vi "Version_4.9_8_on-chip_valves_for25ulSyringe_withModfied_Plunging.vi"() -> ()   [LabVIEW 2020] (continued)
                            n3174 = local read "VISA Refnum in\nfor Pump"() -> (w3578:refnum<visa-resource-name>)
                            n3175 = call "ProcessCompletionWaiter (SubVI).vi"("VISA Refnum in"=w3578) -> ()  [unwired: 11 in]
                          }
                          frame #2 {
                            # "If Yes, it will clean the elution buffer from port-5 tubing a bit more"
                            n3176 = local read "Clean the \nBuffer-B tubing"() -> (w3579:bool)
                            n3177 = case shown="True" w3579 {
                              frame False {
                                n3178 = stacked-sequence {
                                frame #0 {
                                n3179 = local read "Buffer-B Pumping\nResolution"() -> (w3582:T2)
                                n3180 = local read "VISA Refnum in\nfor Pump"() -> (w3584:refnum<visa-resource-name>)
                                n3181 = local read "V-S"() -> (w3581:dbl)
                                n3182 = local read "Volume of Syringe"() -> (w3583:dbl)
                                n3183 = call "RPickUp(SubVI).vi"("Volume to be picked up"=w3581, "Volume of Syringe"=w3583, "Resolution of PickUP"=w3582, "PickUp Flow Rate (ul/min)"=150.0, "VISA Refnum in"=w3584) -> ()  [unwired: 6 in, 1 out]
                                }
                                frame #1 {
                                n3184 = local read "Stopper that ends \nthe main loops"() -> (w3585:bool)
                                n3185 = local read "VISA Refnum in\nfor Pump"() -> (w3586:refnum<visa-resource-name>)
                                n3186 = case shown="True" w3585 {
                                frame False {
                                }
                                frame True {
                                n3187 = local read "VISA Refnum in\nfor Pump"() -> (w3587:refnum<visa-resource-name>)
                                n3188 = call "HardStopCurrentProcess (SubVI).vi"("VISA Refnum in"=w3587) -> ()  [unwired: 11 in]
                                }
                                }
                                n3189 = call "ProcessCompletionWaiter (SubVI).vi"("VISA Refnum in"=w3586) -> ()  [unwired: 11 in]
                                }
                                frame #2 {
                                n3190 = local read "VISA Refnum in\nfor Pump"() -> (w3589:refnum<visa-resource-name>)
                                n3191 = call "PortChanger (SubVI).vi"("Port Number"="1", "VISA Refnum in"=w3589) -> ()  [unwired: 10 in]
                                }
                                frame #3 {
                                n3192 = local read "Stopper that ends \nthe main loops"() -> (w3590:bool)
                                n3193 = local read "VISA Refnum in\nfor Pump"() -> (w3591:refnum<visa-resource-name>)
                                n3194 = case shown="True" w3590 {
                                frame False {
                                }
                                frame True {
                                n3195 = local read "VISA Refnum in\nfor Pump"() -> (w3592:refnum<visa-resource-name>)
                                n3196 = call "HardStopCurrentProcess (SubVI).vi"("VISA Refnum in"=w3592) -> ()  [unwired: 11 in]
                                }
                                }
                                n3197 = call "ProcessCompletionWaiter (SubVI).vi"("VISA Refnum in"=w3591) -> ()  [unwired: 11 in]
                                }
                                frame #4 {
                                n3198 = local read "VISA Refnum in\nfor Pump"() -> (w3597:refnum<visa-resource-name>)
                                n3199 = local read "Volume of Syringe"() -> (w3594:dbl)
                                n3200 = call "GoToAbsolutePosition(SubVI).vi"("Absolute Volume Position in Syringe (in ul)"=0.0, "Volume of Syringe"=w3594, "Resolution of Pumping"=T2."Standard Pumping", "Flow Rate (ul/min)"=150.0, "VISA Refnum in"=w3597) -> ()  [unwired: 6 in, 1 out]
                                }
                                frame #5 {
                                n3201 = local read "Stopper that ends \nthe main loops"() -> (w3598:bool)
                                n3202 = local read "VISA Refnum in\nfor Pump"() -> (w3599:refnum<visa-resource-name>)
                                n3203 = case shown="True" w3598 {
                                frame False {
                                }
                                frame True {
                                n3204 = local read "VISA Refnum in\nfor Pump"() -> (w3600:refnum<visa-resource-name>)
                                n3205 = call "HardStopCurrentProcess (SubVI).vi"("VISA Refnum in"=w3600) -> ()  [unwired: 11 in]
                                }
                                }
                                n3206 = call "ProcessCompletionWaiter (SubVI).vi"("VISA Refnum in"=w3599) -> ()  [unwired: 11 in]
                                }
                                }
                              }
                              frame True {
                                n3207 = for {
                                N: 2 -> [_]
                                n3208 = stacked-sequence {
                                frame #0 {
                                n3209 = local read "Buffer-B Pumping\nResolution"() -> (w3604:T2)
                                n3210 = local read "VISA Refnum in\nfor Pump"() -> (w3606:refnum<visa-resource-name>)
                                n3211 = local read "Apparent Volume\nof Syringe"() -> (w3603:dbl)
                                n3212 = local read "Volume of Syringe"() -> (w3605:dbl)
                                n3213 = call "RPickUp(SubVI).vi"("Volume to be picked up"=w3603, "Volume of Syringe"=w3605, "Resolution of PickUP"=w3604, "PickUp Flow Rate (ul/min)"=150.0, "VISA Refnum in"=w3606) -> ()  [unwired: 6 in, 1 out]
                                }
                                frame #1 {
                                n3214 = local read "Stopper that ends \nthe main loops"() -> (w3607:bool)
                                n3215 = local read "VISA Refnum in\nfor Pump"() -> (w3608:refnum<visa-resource-name>)
                                n3216 = case shown="True" w3607 {
                                frame False {
                                }
                                frame True {
                                n3217 = local read "VISA Refnum in\nfor Pump"() -> (w3609:refnum<visa-resource-name>)
                                n3218 = call "HardStopCurrentProcess (SubVI).vi"("VISA Refnum in"=w3609) -> ()  [unwired: 11 in]
                                }
                                }
                                n3219 = call "ProcessCompletionWaiter (SubVI).vi"("VISA Refnum in"=w3608) -> ()  [unwired: 11 in]
                                }
                                frame #2 {
                                n3220 = local read "VISA Refnum in\nfor Pump"() -> (w3611:refnum<visa-resource-name>)
                                n3221 = call "PortChanger (SubVI).vi"("Port Number"="1", "VISA Refnum in"=w3611) -> ()  [unwired: 10 in]
                                }
                                frame #3 {
                                n3222 = local read "Stopper that ends \nthe main loops"() -> (w3612:bool)
                                n3223 = local read "VISA Refnum in\nfor Pump"() -> (w3613:refnum<visa-resource-name>)
                                n3224 = case shown="True" w3612 {
                                frame False {
                                }
                                frame True {
                                n3225 = local read "VISA Refnum in\nfor Pump"() -> (w3614:refnum<visa-resource-name>)
                                n3226 = call "HardStopCurrentProcess (SubVI).vi"("VISA Refnum in"=w3614) -> ()  [unwired: 11 in]
                                }
                                }
                                n3227 = call "ProcessCompletionWaiter (SubVI).vi"("VISA Refnum in"=w3613) -> ()  [unwired: 11 in]
                                }
                                frame #4 {
                                n3228 = local read "VISA Refnum in\nfor Pump"() -> (w3619:refnum<visa-resource-name>)
                                n3229 = local read "Volume of Syringe"() -> (w3616:dbl)
                                n3230 = call "GoToAbsolutePosition(SubVI).vi"("Absolute Volume Position in Syringe (in ul)"=0.0, "Volume of Syringe"=w3616, "Resolution of Pumping"=T2."Standard Pumping", "Flow Rate (ul/min)"=150.0, "VISA Refnum in"=w3619) -> ()  [unwired: 6 in, 1 out]
                                }
                                frame #5 {
                                n3231 = local read "Stopper that ends \nthe main loops"() -> (w3620:bool)
                                n3232 = local read "VISA Refnum in\nfor Pump"() -> (w3621:refnum<visa-resource-name>)
                                n3233 = case shown="True" w3620 {
                                frame False {
                                }
                                frame True {
                                n3234 = local read "VISA Refnum in\nfor Pump"() -> (w3622:refnum<visa-resource-name>)
                                n3235 = call "HardStopCurrentProcess (SubVI).vi"("VISA Refnum in"=w3622) -> ()  [unwired: 11 in]
                                }
                                }
                                n3236 = call "ProcessCompletionWaiter (SubVI).vi"("VISA Refnum in"=w3621) -> ()  [unwired: 11 in]
                                }
                                }
                                }
                              }
                            }
                          }
                          frame #3 {
                            n3237 = local read "VISA Refnum in\nfor Pump"() -> (w3624:refnum<visa-resource-name>)
                            n3238 = local read "Port for \nB-Elution"() -> (w3623:string)
                            n3239 = call "PortChanger (SubVI).vi"("Port Number"=w3623, "VISA Refnum in"=w3624) -> ()  [unwired: 10 in]
                          }
                          frame #4 {
                            n3240 = local read "VISA Refnum in\nfor Pump"() -> (w3625:refnum<visa-resource-name>)
                            n3241 = call "ProcessCompletionWaiter (SubVI).vi"("VISA Refnum in"=w3625) -> ()  [unwired: 11 in]
                          }
                          frame #5 {
                            n3242 = local read "Buffer-B PickUp \nFlow Rate (ul/min)"() -> (w3628:dbl)
                            n3243 = local read "Buffer-B Pumping\nResolution"() -> (w3627:T2)
                            n3244 = local read "VISA Refnum in\nfor Pump"() -> (w3630:refnum<visa-resource-name>)
                            n3245 = local read "Buffer-B Volume \nto be  Pumped"() -> (w3626:dbl)
                            n3246 = local read "Volume of Syringe"() -> (w3629:dbl)
                            n3247 = call "RPickUp(SubVI).vi"("Volume to be picked up"=w3626, "Volume of Syringe"=w3629, "Resolution of PickUP"=w3627, "PickUp Flow Rate (ul/min)"=w3628, "VISA Refnum in"=w3630) -> ()  [unwired: 6 in, 1 out]
                          }
                          frame #6 {
                            n3248 = local read "Stopper that ends \nthe main loops"() -> (w3631:bool)
                            n3249 = local read "VISA Refnum in\nfor Pump"() -> (w3632:refnum<visa-resource-name>)
                            n3250 = case shown="True" w3631 {
                              frame False {
                              }
                              frame True {
                                n3251 = local read "VISA Refnum in\nfor Pump"() -> (w3633:refnum<visa-resource-name>)
                                n3252 = call "HardStopCurrentProcess (SubVI).vi"("VISA Refnum in"=w3633) -> ()  [unwired: 11 in]
                              }
                            }
                            n3253 = call "ProcessCompletionWaiter (SubVI).vi"("VISA Refnum in"=w3632) -> ()  [unwired: 11 in]
                          }
                          frame #7 {
                            # "Reads the initial Plunger Position for computing the volume dispensed"
                            n3254 = local read "VISA Refnum in\nfor Pump"() -> (w3635:refnum<visa-resource-name>)
                            n3255 = call "AbsolutePlungerPosition (SubVI).vi"("VISA Refnum in"=w3635) -> ("Plunger Position"=w3634:i32)  [unwired: 10 in]
                            n3256 = local write "Initial Plunger Position"(w3634) -> ()
                          }
                          frame #8 {
                            # "Switch to Port-2"
                            # "Port-2 of the pump is conncted to column-1 of chip"
                            n3257 = local read "VISA Refnum in\nfor Pump"() -> (w3637:refnum<visa-resource-name>)
                            n3258 = call "PortChanger (SubVI).vi"("Port Number"="2", "VISA Refnum in"=w3637) -> ()  [unwired: 10 in]
                          }
                          frame #9 {
                            n3259 = local read "Stopper that ends \nthe main loops"() -> (w3638:bool)
                            n3260 = local read "VISA Refnum in\nfor Pump"() -> (w3639:refnum<visa-resource-name>)
                            n3261 = case shown="True" w3638 {
                              frame False {
                              }
                              frame True {
                                n3262 = local read "VISA Refnum in\nfor Pump"() -> (w3640:refnum<visa-resource-name>)
                                n3263 = call "HardStopCurrentProcess (SubVI).vi"("VISA Refnum in"=w3640) -> ()  [unwired: 11 in]
                              }
                            }
                            n3264 = call "ProcessCompletionWaiter (SubVI).vi"("VISA Refnum in"=w3639) -> ()  [unwired: 11 in]
                          }
                          frame #10 {
                            # "Keeps the AMF valve after column-1 open and valve after column-2 closed"
                            n3265 = local read "VISA Refnum in\nfor Valve"() -> (w3645:refnum<visa-resource-name>)
                            n3266 = local read "External Valve \nOPEN"() -> (w3644:string)
                            n3267 = call "PortChanger_Valve (SubVI).vi"("Port Number"=w3644, "VISA Refnum in"=w3645) -> ()  [unwired: 10 in]
                            n3268 = local write "Valve V1 Open"(TRUE ("Valve V1 Open")) -> ()
                            n3269 = local write "Valve V2 Open"(TRUE ("Valve V2 Open")) -> ()
                            n3270 = local write "Valve V3 Open"(FALSE ("Valve V3 Open")) -> ()
                            n3271 = local write "Valve V4 Open"(FALSE ("Valve V4 Open")) -> ()
                            n3272 = local write "Valve V6 Open"(FALSE ("Valve V6 Open")) -> ()
                            n3273 = local write "Valve V5 Open"(FALSE ("Valve V5 Open")) -> ()
                            n3274 = local write "Valve V7 Open"(FALSE ("Valve V7 Open")) -> ()
                          }
                          frame #11 {
                            n3275 = local read "Buffer-B Dispense\nFlow Rate (ul/min)"() -> (w3655:dbl)
                            n3276 = local read "Buffer-B Pumping\nResolution"() -> (w3654:T2)
                            n3277 = local read "Initial Plunger Position"() -> (w3651:dbl)
                            n3278 = local read "VISA Refnum in\nfor Pump"() -> (w3657:refnum<visa-resource-name>)
                            n3279 = local read "Volume of Syringe"() -> (w3656:dbl)
                            n3280 = call "GoToAbsolutePosition(SubVI).vi"("Absolute Volume Position in Syringe (in ul)"=0.0 ("Volume to be Dispensed"), "Volume of Syringe"=w3656, "Resolution of Pumping"=w3654, "Flow Rate (ul/min)"=w3655, "VISA Refnum in"=w3657) -> ()  [unwired: 6 in, 1 out]
                            n3281 = local write "Pause Data Collection"(FALSE ("Pause Data Collection")) -> ()
                            n3282 = local write "Vol_now"(0.0 ("Vol_now")) -> ()
                            n3283 = local write "Position\nNow"(w3651) -> ()
                          }
                          frame #12 {
                            n3284 = while {
                              stop <- w3664 stop-if-true
                              n3285 = event shown="[0] \"Pause Elution Value\": Value Change" {
                                selector: _ -> [_ _]
                                dyn-events: _ -> [_ _]
                                timeout: 100 -> [_ _]
                                event "Pause Elution\nValue": Value Change {
                                n3286 = event-data() -> ()  [unwired: 1 in, 6 out]
                                n3287 = stacked-sequence {
                                frame #0 {
                                n3288 = local read "Pause Elution"() -> (w3666:bool)
                                n3289 = case shown="False" w3666 {
                                frame False {
                                n3290 = local write "Pause Elution"(TRUE ("Pause Elution")) -> ()
                                }
                                frame True {
                                n3291 = local write "Pause Elution"(FALSE ("Pause Elution")) -> ()
                                }
                                }
                                }
                                frame #1 {
                                n3292 = local read "Pause Elution"() -> (w3669:bool)
                                n3293 = case shown="False" w3669 {
                                frame False {
                                n3294 = local read "Buffer-B Dispense\nFlow Rate (ul/min)"() -> (w3674:dbl)
                                n3295 = local read "VISA Refnum in\nfor Pump"() -> (w3675:refnum<visa-resource-name>)
                                n3296 = local read "Buffer-B Pumping\nResolution"() -> (w3671:T2)
                                n3297 = local read "Volume of Syringe"() -> (w3672:dbl)
                                n3298 = call "GoToAbsolutePosition(SubVI).vi"("Absolute Volume Position in Syringe (in ul)"=0.0, "Volume of Syringe"=w3672, "Resolution of Pumping"=w3671, "Flow Rate (ul/min)"=w3674, "VISA Refnum in"=w3675) -> ()  [unwired: 6 in, 1 out]
                                n3299 = local write "Pause Data Collection"(FALSE ("Pause Data Collection")) -> ()
                                }
                                frame True {
                                n3300 = local read "VISA Refnum in\nfor Pump"() -> (w3677:refnum<visa-resource-name>)
                                n3301 = local write "Pause Data Collection"(TRUE ("Pause Data Collection")) -> ()
                                n3302 = call "HardStopCurrentProcess (SubVI).vi"("VISA Refnum in"=w3677) -> ()  [unwired: 11 in]
                                }
                                }
                                }
                                }
                                }
                                event Timeout {
                                n3303 = event-data() -> ()  [unwired: 1 in, 3 out]
                                }
                              }
                              n3304 = local read "Divert Sample \ninto Column-2"() -> (w3663:bool)
                              n3305 = local read "Stopper that ends \nthe main loops"() -> (w3662:bool)
                              n3306 = Or(x=w3663, y=w3662) -> (x .or. y?=w3664:bool)
                            }
                            n3307 = local read "Buffer-B Pumping\nResolution"() -> (w3660:T2)
                            n3308 = local read "VISA Refnum in\nfor Pump"() -> (w3661:refnum<visa-resource-name>)
                            n3309 = local read "Volume of Syringe"() -> (w3659:dbl)
                            n3310 = while {
                              tunnel: w3661 -> [w3686]
                              tunnel: w3660 -> [w3685]
                              tunnel: w3659 -> [w3684]
                              stop <- w3680 stop-if-true
                              n3311 = local read "Position\nNow"() -> (w3678:dbl)
                              n3312 = local read "Pause Elution"() -> (w3679:bool)
                              n3313 = case shown="True" w3679 {
                                tunnel: w3678 -> [w3690 _]
                                tunnel: w3686 -> [w3689 w3732]
                                tunnel: w3685 -> [w3688 _]
                                tunnel: w3684 -> [w3687 _]
                                frame False {
                                n3314 = stacked-sequence {
                                tunnel: w3690 -> [_ w3696]
                                tunnel: w3689 -> [_ w3695]
                                tunnel: w3688 -> [_ w3694]
                                tunnel: w3687 -> [_ w3693]
                                frame #0 {
                                n3315 = Wait (ms)(milliseconds to wait=u32 3000) -> ()  [unwired: 1 out]
                                n3316 = local write "Signal"(TRUE ("Signal")) -> ()
                                }
                                frame #1 {
                                n3317 = while {
                                tunnel: w3696 -> [w3708]
                                tunnel: w3695 -> [w3707]
                                tunnel: w3694 -> [w3706]
                                tunnel: w3693 -> [w3705]
                                stop <- w3700 stop-if-true
                                n3318 = stacked-sequence {
                                tunnel: w3708 -> [_ w3715]
                                tunnel: w3707 -> [_ w3714]
                                tunnel: w3706 -> [_ w3713]
                                tunnel: w3705 -> [_ w3712]
                                frame #0 {
                                n3319 = Wait (ms)(milliseconds to wait=u32 500) -> ()  [unwired: 1 out]
                                }
                                frame #1 {
                                n3320 = call "AbsolutePlungerPosition (SubVI).vi"("VISA Refnum in"=w3714) -> ("Plunger Position"=w3711:i32)  [unwired: 10 in]
                                n3321 = case shown="\"High Resolution Pumping\"" w3713 {
                                tunnel: w3715 -> [w3720 w3729]
                                tunnel: w3711 -> [w3721 w3728]
                                tunnel: [w3719 w3726] -> w3710
                                tunnel: w3712 -> [w3718 w3727]
                                frame "Standard Pumping", Default {
                                n3322 = Subtract(x=w3720, y=w3721) -> (x-y=w3717:dbl)
                                n3323 = Absolute Value(x=w3717) -> (abs(x)=w3716:dbl)
                                n3324 = Multiply(x=w3716, y=w3718) -> (x*y=w3723:dbl)
                                n3325 = Divide(x=w3723, y=3000.0) -> (x/y=w3719:dbl)
                                }
                                frame "High Resolution Pumping" {
                                n3326 = Subtract(x=w3729, y=w3728) -> (x-y=w3725:dbl)
                                n3327 = Absolute Value(x=w3725) -> (abs(x)=w3724:dbl)
                                n3328 = Multiply(x=w3724, y=w3727) -> (x*y=w3731:dbl)
                                n3329 = Divide(x=w3731, y=24000.0) -> (x/y=w3726:dbl)
                                }
                                }
                                n3330 = local write "Volume being Injected \nin this process"(w3710) -> ()
                                }
                                }
                                n3331 = local read "Volume being Injected \nin this process"() -> (w3698:dbl)
                                n3332 = local read "Affinity Elution \nGraph Min CutOff"() -> (w3697:dbl)
                                n3333 = local read "Stopper that ends \nthe main loops"() -> (w3703:bool)
                                n3334 = local read "Divert Sample \ninto Column-2"() -> (w3704:bool)
                                n3335 = Greater Or Equal?(x=w3698, y=w3697) -> (x >= y?=w3699:bool)
                                n3336 = Or(x=w3704, y=w3703) -> (x .or. y?=w3701:bool)
                                n3337 = local read "Pause Elution"() -> (w3702:bool)
                                n3338 = local write "Affinity Elution \nis Approaching"(w3699) -> ()
                                n3339 = Or(x=w3702, y=w3701) -> (x .or. y?=w3700:bool)
                                }
                                }
                                }
                                }
                                frame True {
                                n3340 = stacked-sequence {
                                tunnel: w3732 -> [_ w3735 _]
                                frame #0 {
                                n3341 = Wait (ms)(milliseconds to wait=u32 2000) -> ()  [unwired: 1 out]
                                }
                                frame #1 {
                                n3342 = local read "Signal"() -> (w3734:bool)
                                n3343 = case shown="True" w3734 {
                                tunnel: w3735 -> [_ w3741]
                                frame False {
                                }
                                frame True {
                                n3344 = local read "Volume being Injected \nin this process"() -> (w3739:dbl)
                                n3345 = local read "Net Elution \nVolume"() -> (w3738:dbl)
                                n3346 = local write "Signal"(FALSE ("Signal")) -> ()
                                n3347 = Add(x=w3739, y=w3738) -> (x+y=w3737:dbl)
                                n3348 = call "AbsolutePlungerPosition (SubVI).vi"("VISA Refnum in"=w3741) -> ("Plunger Position"=w3740:i32)  [unwired: 10 in]
                                n3349 = local write "Net Elution \nVolume"(w3737) -> ()
                                n3350 = local write "Position\nNow"(w3740) -> ()
                                }
                                }
                                }
                                frame #2 {
                                n3351 = local write "Volume being Injected \nin this process"(0.0 ("Volume being Injected \nin this process")) -> ()
                                }
                                }
                                }
                              }
                              n3352 = local read "Stopper that ends \nthe main loops"() -> (w3682:bool)
                              n3353 = local read "Divert Sample \ninto Column-2"() -> (w3681:bool)
                              n3354 = Or(x=w3681, y=w3682) -> (x .or. y?=w3680:bool)
                              n3355 = Wait (ms)(milliseconds to wait=u32 300) -> ()  [unwired: 1 out]
                            }
                            n3356 = local read "Stopper that ends \nthe main loops"() -> (w3658:bool)
                            n3357 = case shown="True" w3658 {
                              frame False {
                              }
                              frame True {
                                n3358 = local read "VISA Refnum in\nfor Pump"() -> (w3743:refnum<visa-resource-name>)
                                n3359 = call "HardStopCurrentProcess (SubVI).vi"("VISA Refnum in"=w3743) -> ()  [unwired: 11 in]
                              }
                            }
                          }
                          frame #13 {
                            # "valve after column-1 is closed"
                            # "Keeps the on-chip Valve V1 and V3 after column-2 open"
                            # "Keeps the AMF valve after column-1 closed and valve after column-2 open"
                            n3360 = local read "VISA Refnum in\nfor Pump"() -> (w3756:refnum<visa-resource-name>)
                            n3361 = local read "Volume being Injected \nin this process"() -> (w3753:dbl)
                            n3362 = local write "Sample Volume Diverted\ninto Column-2"(0.0 ("Sample Volume Diverted\ninto Column-2")) -> ()
                            n3363 = call "AbsolutePlungerPosition (SubVI).vi"("VISA Refnum in"=w3756) -> ("Plunger Position"=w3755:i32)  [unwired: 10 in]
                            n3364 = local write "Position\nNow"(w3755) -> ()
                            n3365 = local write "Vol_previous"(0.0 ("Vol_diff")) -> ()
                            n3366 = local write "Vol_now"(w3753) -> ()
                            n3367 = local read "VISA Refnum in\nfor Valve"() -> (w3748:refnum<visa-resource-name>)
                            n3368 = local read "External Valve \nCLOSED"() -> (w3747:string)
                            n3369 = local write "Valve V1 Open"(TRUE ("Valve V1 Open")) -> ()
                            n3370 = local write "Valve V3 Open"(TRUE ("Valve V3 Open")) -> ()
                            n3371 = local write "Valve V2 Open"(FALSE ("Valve V2 Open")) -> ()
                            n3372 = local write "Valve V4 Open"(TRUE ("Valve V4 Open")) -> ()
                            n3373 = call "PortChanger_Valve (SubVI).vi"("Port Number"=w3747, "VISA Refnum in"=w3748) -> ()  [unwired: 10 in]
                            n3374 = local write "Valve V5 Open"(TRUE ("Valve V5 Open")) -> ()
                            n3375 = local write "Valve V6 Open"(FALSE ("Valve V6 Open")) -> ()
                            n3376 = local write "Valve V7 Open"(TRUE ("Valve V7 Open")) -> ()
                          }
                          frame #14 {
                            n3377 = local read "Divert Sample \ninto Column-2"() -> (w3758:bool)
                            n3378 = case shown="True" w3758 {
                              frame False {
                                n3379 = stacked-sequence {
                                frame #0 {
                                n3380 = local read "Buffer-B Pumping\nResolution"() -> (w3761:T2)
                                n3381 = local read "VISA Refnum in\nfor Pump"() -> (w3763:refnum<visa-resource-name>)
                                n3382 = local read "Initial Plunger Position"() -> (w3762:dbl)
                                n3383 = local read "Volume of Syringe"() -> (w3760:dbl)
                                n3384 = while {
                                tunnel: w3762 -> [w3769]
                                tunnel: w3763 -> [w3768]
                                tunnel: w3761 -> [w3767]
                                tunnel: w3760 -> [w3766]
                                stop <- w3764 stop-if-true
                                n3385 = Wait (ms)(milliseconds to wait=u32 100) -> ()  [unwired: 1 out]
                                n3386 = stacked-sequence {
                                tunnel: w3769 -> [w3775 _]
                                tunnel: w3768 -> [w3774 w3795]
                                tunnel: w3767 -> [w3773 _]
                                tunnel: w3766 -> [w3772 _]
                                tunnel: [_ w3793] -> w3764
                                frame #0 {
                                n3387 = call "AbsolutePlungerPosition (SubVI).vi"("VISA Refnum in"=w3774) -> ("Plunger Position"=w3771:i32)  [unwired: 10 in]
                                n3388 = case shown="\"Standard Pumping\", Default" w3773 {
                                tunnel: w3775 -> [w3780 w3789]
                                tunnel: w3771 -> [w3781 w3788]
                                tunnel: [w3779 w3786] -> w3770
                                tunnel: w3772 -> [w3778 w3787]
                                frame "Standard Pumping", Default {
                                n3389 = Subtract(x=w3780, y=w3781) -> (x-y=w3777:dbl)
                                n3390 = Absolute Value(x=w3777) -> (abs(x)=w3776:dbl)
                                n3391 = Multiply(x=w3776, y=w3778) -> (x*y=w3783:dbl)
                                n3392 = Divide(x=w3783, y=3000.0) -> (x/y=w3779:dbl)
                                }
                                frame "High Resolution Pumping" {
                                n3393 = Subtract(x=w3789, y=w3788) -> (x-y=w3785:dbl)
                                n3394 = Absolute Value(x=w3785) -> (abs(x)=w3784:dbl)
                                n3395 = Multiply(x=w3784, y=w3787) -> (x*y=w3791:dbl)
                                n3396 = Divide(x=w3791, y=24000.0) -> (x/y=w3786:dbl)
                                }
                                }
                                n3397 = local write "Volume being Injected \nin this process"(w3770) -> ()
                                }
                                frame #1 {
                                n3398 = local read "Stopper that ends \nthe main loops"() -> (w3792:bool)
                                n3399 = call "LSPOneStatus (SubVI).vi"("VISA Refnum in"=w3795) -> ("read buffer"=w3797:string)  [unwired: 10 in]
                                n3400 = call <vilib>:"Trim Whitespace.vi"("string"=w3797) -> ("trimmed string"=w3796:string)  [unwired: 1 in]
                                n3401 = Equal?(x=w3796, y="/0`\u0003") -> (x = y?=w3794:bool)
                                n3402 = Or(x=w3794, y=w3792) -> (x .or. y?=w3793:bool)
                                }
                                }
                                }
                                n3403 = local read "Stopper that ends \nthe main loops"() -> (w3759:bool)
                                n3404 = case shown="True" w3759 {
                                frame False {
                                }
                                frame True {
                                n3405 = local read "VISA Refnum in\nfor Pump"() -> (w3799:refnum<visa-resource-name>)
                                n3406 = call "HardStopCurrentProcess (SubVI).vi"("VISA Refnum in"=w3799) -> ()  [unwired: 11 in]
                                }
                                }
                                }
                                }
                              }
                              frame True {
                                n3407 = stacked-sequence {
                                frame #0 {
                                n3408 = local read "Buffer-B Pumping\nResolution"() -> (w3802:T2)
                                n3409 = local read "VISA Refnum in\nfor Pump"() -> (w3804:refnum<visa-resource-name>)
                                n3410 = local read "Volume of Syringe"() -> (w3801:dbl)
                                n3411 = local read "Position\nNow"() -> (w3803:dbl)
                                n3412 = while {
                                tunnel: w3803 -> [w3810]
                                tunnel: w3804 -> [w3809]
                                tunnel: w3802 -> [w3808]
                                tunnel: w3801 -> [w3807]
                                stop <- w3805 stop-if-true
                                n3413 = Wait (ms)(milliseconds to wait=u32 100) -> ()  [unwired: 1 out]
                                n3414 = stacked-sequence {
                                tunnel: w3810 -> [w3820 _ _]
                                tunnel: w3809 -> [w3819 _ w3846]
                                tunnel: w3808 -> [w3818 _ _]
                                tunnel: w3807 -> [w3817 _ _]
                                tunnel: [_ _ w3844] -> w3805
                                frame #0 {
                                n3415 = local read "Vol_previous"() -> (w3814:dbl)
                                n3416 = call "AbsolutePlungerPosition (SubVI).vi"("VISA Refnum in"=w3819) -> ("Plunger Position"=w3816:i32)  [unwired: 10 in]
                                n3417 = case shown="\"Standard Pumping\", Default" w3818 {
                                tunnel: w3820 -> [w3825 w3834]
                                tunnel: w3816 -> [w3826 w3833]
                                tunnel: [w3824 w3831] -> w3815
                                tunnel: w3817 -> [w3823 w3832]
                                frame "Standard Pumping", Default {
                                n3418 = Subtract(x=w3825, y=w3826) -> (x-y=w3822:dbl)
                                n3419 = Absolute Value(x=w3822) -> (abs(x)=w3821:dbl)
                                n3420 = Multiply(x=w3821, y=w3823) -> (x*y=w3828:dbl)
                                n3421 = Divide(x=w3828, y=3000.0) -> (x/y=w3824:dbl)
                                }
                                frame "High Resolution Pumping" {
                                n3422 = Subtract(x=w3834, y=w3833) -> (x-y=w3830:dbl)
                                n3423 = Absolute Value(x=w3830) -> (abs(x)=w3829:dbl)
                                n3424 = Multiply(x=w3829, y=w3832) -> (x*y=w3836:dbl)
                                n3425 = Divide(x=w3836, y=24000.0) -> (x/y=w3831:dbl)
                                }
                                }
                                n3426 = Subtract(x=w3815, y=w3814) -> (x-y=w3813:dbl)
                                n3427 = local read "Vol_now"() -> (w3811:dbl)
                                n3428 = local write "Sample Volume Diverted\ninto Column-2"(w3815) -> ()
                                n3429 = Add(x=w3813, y=w3811) -> (x+y=w3812:dbl)
                                n3430 = local write "Volume being Injected \nin this process"(w3812) -> ()
                                }
                                frame #1 {
                                n3431 = local read "Volume being Injected \nin this process"() -> (w3837:dbl)
                                n3432 = local read "Sample Volume Diverted\ninto Column-2"() -> (w3838:dbl)
                                n3433 = local write "Vol_now"(w3837) -> ()
                                n3434 = local write "Vol_previous"(w3838) -> ()
                                }
                                frame #2 {
                                n3435 = local read "Buffer-B Volume \nto be Pumped for\nSample Diversion\nto Column-2"() -> (w3840:dbl)
                                n3436 = local read "Sample Volume Diverted\ninto Column-2"() -> (w3839:dbl)
                                n3437 = local read "Stopper that ends \nthe main loops"() -> (w3841:bool)
                                n3438 = call "LSPOneStatus (SubVI).vi"("VISA Refnum in"=w3846) -> ("read buffer"=w3848:string)  [unwired: 10 in]
                                n3439 = call <vilib>:"Trim Whitespace.vi"("string"=w3848) -> ("trimmed string"=w3847:string)  [unwired: 1 in]
                                n3440 = Equal?(x=w3847, y="/0`\u0003") -> (x = y?=w3845:bool)
                                n3441 = Greater Or Equal?(x=w3839, y=w3840) -> (x >= y?=w3843:bool)
                                n3442 = Or(x=w3841, y=w3843) -> (x .or. y?=w3842:bool)
                                n3443 = Or(x=w3845, y=w3842) -> (x .or. y?=w3844:bool)
                                }
                                }
                                }
                                n3444 = local read "Stopper that ends \nthe main loops"() -> (w3800:bool)
                                n3445 = case shown="True" w3800 {
                                frame False {
                                }
                                frame True {
                                n3446 = local read "VISA Refnum in\nfor Pump"() -> (w3850:refnum<visa-resource-name>)
                                n3447 = call "HardStopCurrentProcess (SubVI).vi"("VISA Refnum in"=w3850) -> ()  [unwired: 11 in]
                                }
                                }
                                }
                                frame #1 {
                                n3448 = local read "VISA Refnum in\nfor Pump"() -> (w3852:refnum<visa-resource-name>)
                                n3449 = local write "Pause Data Collection"(TRUE ("Pause Data Collection")) -> ()
                                n3450 = call "HardStopCurrentProcess (SubVI).vi"("VISA Refnum in"=w3852) -> ()  [unwired: 11 in]
                                }
                                frame #2 {
                                n3451 = local read "VISA Refnum in\nfor Pump"() -> (w3853:refnum<visa-resource-name>)
                                n3452 = call "PortChanger (SubVI).vi"("Port Number"="1", "VISA Refnum in"=w3853) -> ()  [unwired: 10 in]
                                }
                                frame #3 {
                                n3453 = local read "VISA Refnum in\nfor Pump"() -> (w3859:refnum<visa-resource-name>)
                                n3454 = local read "Volume of Syringe"() -> (w3855:dbl)
                                n3455 = call "GoToAbsolutePosition(SubVI).vi"("Absolute Volume Position in Syringe (in ul)"=0.0, "Volume of Syringe"=w3855, "Resolution of Pumping"=T2."Standard Pumping", "Flow Rate (ul/min)"=150.0, "VISA Refnum in"=w3859) -> ()  [unwired: 6 in, 1 out]
                                }
                                frame #4 {
                                n3456 = local read "VISA Refnum in\nfor Pump"() -> (w3861:refnum<visa-resource-name>)
                                n3457 = local write "Divert Sample \ninto Column-2"(FALSE ("Divert Sample \ninto Column-2")) -> ()
                                n3458 = call "ProcessCompletionWaiter (SubVI).vi"("VISA Refnum in"=w3861) -> ()  [unwired: 11 in]
                                }
                                }
                              }
                            }
                          }
                          frame #15 {
                            # "Keeps the On-Chip Valves V1 and V3 closed"
                            # "Switch to Port-5/8"
                            # "Port-5/8 of pump is connected to Buffer-C1/C2"
                            # "Keeps the AMF valve after column-1 open and valve after column-2 closed"
                            n3459 = local read "VISA Refnum in\nfor Pump"() -> (w3874:refnum<visa-resource-name>)
                            n3460 = local write "Pause Data Collection"(TRUE ("Pause Data Collection")) -> ()
                            n3461 = Wait (ms)(milliseconds to wait=u32 500) -> ()  [unwired: 1 out]
                            n3462 = local write "Affinity On"(FALSE ("Affinity On")) -> ()
                            n3463 = local read "Port for \nC2-Elution"() -> (w3865:string)
                            n3464 = local write "Affinity Elution On"(FALSE ("Affinity Elution On")) -> ()
                            n3465 = call "PortChanger (SubVI).vi"("Port Number"=w3865, "VISA Refnum in"=w3874) -> ()  [unwired: 10 in]
                            n3466 = local read "VISA Refnum in\nfor Valve"() -> (w3868:refnum<visa-resource-name>)
                            n3467 = local read "External Valve \nCLOSED"() -> (w3867:string)
                            n3468 = local write "Valve V1 Open"(FALSE ("Valve V1 Open")) -> ()
                            n3469 = local write "Valve V2 Open"(FALSE ("Valve V2 Open")) -> ()
                            n3470 = local write "Valve V3 Open"(FALSE ("Valve V3 Open")) -> ()
                            n3471 = local write "Valve V4 Open"(FALSE ("Valve V4 Open")) -> ()
                            n3472 = call "PortChanger_Valve (SubVI).vi"("Port Number"=w3867, "VISA Refnum in"=w3868) -> ()  [unwired: 10 in]
                            n3473 = local write "Valve V5 Open"(FALSE ("Valve V5 Open")) -> ()
                            n3474 = local write "Valve V6 Open"(FALSE ("Valve V6 Open")) -> ()
                            n3475 = local write "Valve V7 Open"(FALSE ("Valve V7 Open")) -> ()
                          }
                          frame #16 {
                            n3476 = local read "VISA Refnum in\nfor Pump"() -> (w3878:refnum<visa-resource-name>)
                            n3477 = call "ProcessCompletionWaiter (SubVI).vi"("VISA Refnum in"=w3878) -> ()  [unwired: 11 in]
                            n3478 = local write "Start the Process"(FALSE ("Start the Process")) -> ()
                          }
                          frame #17 {
                            n3479 = local read "Stopper that ends \nthe main loops"() -> (w3882:bool)
                            n3480 = local read "Start the Process"() -> (w3883:bool)
                            n3481 = Or(x=w3883, y=w3882) -> (x .or. y?=w3881:bool)
                            n3482 = local write "Elution of Column-1"(FALSE ("Elution of Column-1")) -> ()
                            n3483 = case shown="False" w3881 {
                              frame False {
                                n3484 = while {
                                stop <- w3887 stop-if-true
                                n3485 = local read "Stopper that ends \nthe main loops"() -> (w3888:bool)
                                n3486 = local read "Start the Process"() -> (w3889:bool)
                                n3487 = Or(x=w3889, y=w3888) -> (x .or. y?=w3887:bool)
                                n3488 = Wait (ms)(milliseconds to wait=u32 10) -> ()  [unwired: 1 out]
                                }
                                n3489 = One Button Dialog(message="Move to Column-2 detection zone and Press 'Start the Process' Button.") -> ()  [unwired: 1 in, 1 out]
                              }
                              frame True {
                              }
                            }
                            n3490 = local write "Volume being Injected \nin this process"(0.0 ("Volume being Injected \nin this process")) -> ()
                            n3491 = local write "Elution of Column-2"(TRUE ("Elution of Column-2")) -> ()
                          }
                          frame #18 {
                            # "If Yes, it will clean the SEC buffer from port-8 tubing else it will clean the pump valve a bit"
                            n3492 = local read "Clean the \nBuffer-C2 tubing"() -> (w3890:bool)
                            n3493 = case shown="False" w3890 {
                              frame False {
                                n3494 = stacked-sequence {
                                frame #0 {
                                n3495 = local read "VISA Refnum in\nfor Pump"() -> (w3892:refnum<visa-resource-name>)
                                n3496 = local read "Port for \nC2-Elution"() -> (w3891:string)
                                n3497 = call "PortChanger (SubVI).vi"("Port Number"=w3891, "VISA Refnum in"=w3892) -> ()  [unwired: 10 in]
                                }
                                frame #1 {
                                n3498 = local read "VISA Refnum in\nfor Pump"() -> (w3893:refnum<visa-resource-name>)
                                n3499 = call "ProcessCompletionWaiter (SubVI).vi"("VISA Refnum in"=w3893) -> ()  [unwired: 11 in]
                                }
                                frame #2 {
                                n3500 = local read "Buffer-C2 Pumping\nResolution"() -> (w3896:T2)
                                n3501 = local read "VISA Refnum in\nfor Pump"() -> (w3898:refnum<visa-resource-name>)
                                n3502 = local read "V-S"() -> (w3894:dbl)
                                n3503 = local read "Volume of Syringe"() -> (w3897:dbl)
                                n3504 = call "RPickUp(SubVI).vi"("Volume to be picked up"=w3894, "Volume of Syringe"=w3897, "Resolution of PickUP"=w3896, "PickUp Flow Rate (ul/min)"=150.0, "VISA Refnum in"=w3898) -> ()  [unwired: 6 in, 1 out]
                                }
                                frame #3 {
                                n3505 = local read "Stopper that ends \nthe main loops"() -> (w3899:bool)
                                n3506 = local read "VISA Refnum in\nfor Pump"() -> (w3900:refnum<visa-resource-name>)
                                n3507 = case shown="True" w3899 {
                                frame False {
                                }
                                frame True {
                                n3508 = local read "VISA Refnum in\nfor Pump"() -> (w3901:refnum<visa-resource-name>)
                                n3509 = call "HardStopCurrentProcess (SubVI).vi"("VISA Refnum in"=w3901) -> ()  [unwired: 11 in]
                                }
                                }
                                n3510 = call "ProcessCompletionWaiter (SubVI).vi"("VISA Refnum in"=w3900) -> ()  [unwired: 11 in]
                                }
                                frame #4 {
                                n3511 = local read "VISA Refnum in\nfor Pump"() -> (w3903:refnum<visa-resource-name>)
                                n3512 = call "PortChanger (SubVI).vi"("Port Number"="1", "VISA Refnum in"=w3903) -> ()  [unwired: 10 in]
                                }
                                frame #5 {
                                n3513 = local read "Stopper that ends \nthe main loops"() -> (w3904:bool)
                                n3514 = local read "VISA Refnum in\nfor Pump"() -> (w3905:refnum<visa-resource-name>)
                                n3515 = case shown="True" w3904 {
                                frame False {
                                }
                                frame True {
                                n3516 = local read "VISA Refnum in\nfor Pump"() -> (w3906:refnum<visa-resource-name>)
                                n3517 = call "HardStopCurrentProcess (SubVI).vi"("VISA Refnum in"=w3906) -> ()  [unwired: 11 in]
                                }
                                }
                                n3518 = call "ProcessCompletionWaiter (SubVI).vi"("VISA Refnum in"=w3905) -> ()  [unwired: 11 in]
                                }
                                frame #6 {
                                n3519 = local read "VISA Refnum in\nfor Pump"() -> (w3911:refnum<visa-resource-name>)
                                n3520 = local read "Volume of Syringe"() -> (w3908:dbl)
                                n3521 = call "GoToAbsolutePosition(SubVI).vi"("Absolute Volume Position in Syringe (in ul)"=0.0, "Volume of Syringe"=w3908, "Resolution of Pumping"=T2."Standard Pumping", "Flow Rate (ul/min)"=150.0, "VISA Refnum in"=w3911) -> ()  [unwired: 6 in, 1 out]
                                }
                                frame #7 {
                                n3522 = local read "Stopper that ends \nthe main loops"() -> (w3912:bool)
                                n3523 = local read "VISA Refnum in\nfor Pump"() -> (w3913:refnum<visa-resource-name>)
                                n3524 = case shown="True" w3912 {
                                frame False {
                                }
                                frame True {
                                n3525 = local read "VISA Refnum in\nfor Pump"() -> (w3914:refnum<visa-resource-name>)
                                n3526 = call "HardStopCurrentProcess (SubVI).vi"("VISA Refnum in"=w3914) -> ()  [unwired: 11 in]
                                }
                                }
                                n3527 = call "ProcessCompletionWaiter (SubVI).vi"("VISA Refnum in"=w3913) -> ()  [unwired: 11 in]
                                }
                                }
                              }
                              frame True {
                                n3528 = for {
                                N: 2 -> [_]
                                n3529 = stacked-sequence {
                                frame #0 {
                                n3530 = local read "VISA Refnum in\nfor Pump"() -> (w3917:refnum<visa-resource-name>)
                                n3531 = local read "Port for \nC2-Elution"() -> (w3916:string)
                                n3532 = call "PortChanger (SubVI).vi"("Port Number"=w3916, "VISA Refnum in"=w3917) -> ()  [unwired: 10 in]
                                }
                                frame #1 {
                                n3533 = local read "VISA Refnum in\nfor Pump"() -> (w3918:refnum<visa-resource-name>)
                                n3534 = call "ProcessCompletionWaiter (SubVI).vi"("VISA Refnum in"=w3918) -> ()  [unwired: 11 in]
                                }
                                frame #2 {
                                n3535 = local read "Buffer-C2 Pumping\nResolution"() -> (w3921:T2)
                                n3536 = local read "VISA Refnum in\nfor Pump"() -> (w3923:refnum<visa-resource-name>)
                                n3537 = local read "Apparent Volume\nof Syringe"() -> (w3919:dbl)
                                n3538 = local read "Volume of Syringe"() -> (w3922:dbl)
                                n3539 = call "RPickUp(SubVI).vi"("Volume to be picked up"=w3919, "Volume of Syringe"=w3922, "Resolution of PickUP"=w3921, "PickUp Flow Rate (ul/min)"=150.0, "VISA Refnum in"=w3923) -> ()  [unwired: 6 in, 1 out]
                                }
                                frame #3 {
                                n3540 = local read "Stopper that ends \nthe main loops"() -> (w3924:bool)
                                n3541 = local read "VISA Refnum in\nfor Pump"() -> (w3925:refnum<visa-resource-name>)
                                n3542 = case shown="True" w3924 {
                                frame False {
                                }
                                frame True {
                                n3543 = local read "VISA Refnum in\nfor Pump"() -> (w3926:refnum<visa-resource-name>)
                                n3544 = call "HardStopCurrentProcess (SubVI).vi"("VISA Refnum in"=w3926) -> ()  [unwired: 11 in]
                                }
                                }
                                n3545 = call "ProcessCompletionWaiter (SubVI).vi"("VISA Refnum in"=w3925) -> ()  [unwired: 11 in]
                                }
                                frame #4 {
                                n3546 = local read "VISA Refnum in\nfor Pump"() -> (w3928:refnum<visa-resource-name>)
                                n3547 = call "PortChanger (SubVI).vi"("Port Number"="1", "VISA Refnum in"=w3928) -> ()  [unwired: 10 in]
                                }
                                frame #5 {
                                n3548 = local read "Stopper that ends \nthe main loops"() -> (w3929:bool)
                                n3549 = local read "VISA Refnum in\nfor Pump"() -> (w3930:refnum<visa-resource-name>)
                                n3550 = case shown="True" w3929 {
                                frame False {
                                }
                                frame True {
                                n3551 = local read "VISA Refnum in\nfor Pump"() -> (w3931:refnum<visa-resource-name>)
                                n3552 = call "HardStopCurrentProcess (SubVI).vi"("VISA Refnum in"=w3931) -> ()  [unwired: 11 in]
                                }
                                }
                                n3553 = call "ProcessCompletionWaiter (SubVI).vi"("VISA Refnum in"=w3930) -> ()  [unwired: 11 in]
                                }
                                frame #6 {
                                n3554 = local read "VISA Refnum in\nfor Pump"() -> (w3936:refnum<visa-resource-name>)
                                n3555 = local read "Volume of Syringe"() -> (w3933:dbl)
                                n3556 = call "GoToAbsolutePosition(SubVI).vi"("Absolute Volume Position in Syringe (in ul)"=0.0, "Volume of Syringe"=w3933, "Resolution of Pumping"=T2."Standard Pumping", "Flow Rate (ul/min)"=150.0, "VISA Refnum in"=w3936) -> ()  [unwired: 6 in, 1 out]
                                }
                                frame #7 {
                                n3557 = local read "Stopper that ends \nthe main loops"() -> (w3937:bool)
                                n3558 = local read "VISA Refnum in\nfor Pump"() -> (w3938:refnum<visa-resource-name>)
                                n3559 = case shown="True" w3937 {
                                frame False {
                                }
                                frame True {
                                n3560 = local read "VISA Refnum in\nfor Pump"() -> (w3939:refnum<visa-resource-name>)
                                n3561 = call "HardStopCurrentProcess (SubVI).vi"("VISA Refnum in"=w3939) -> ()  [unwired: 11 in]
                                }
                                }
                                n3562 = call "ProcessCompletionWaiter (SubVI).vi"("VISA Refnum in"=w3938) -> ()  [unwired: 11 in]
                                }
                                }
                                }
                              }
                            }
                          }
                          frame #19 {
                            n3563 = local read "VISA Refnum in\nfor Pump"() -> (w3941:refnum<visa-resource-name>)
                            n3564 = local read "Port for \nC2-Elution"() -> (w3940:string)
                            n3565 = call "PortChanger (SubVI).vi"("Port Number"=w3940, "VISA Refnum in"=w3941) -> ()  [unwired: 10 in]
                          }
                          frame #20 {
                            n3566 = local read "VISA Refnum in\nfor Pump"() -> (w3942:refnum<visa-resource-name>)
                            n3567 = call "ProcessCompletionWaiter (SubVI).vi"("VISA Refnum in"=w3942) -> ()  [unwired: 11 in]
                          }
                          frame #21 {
                            n3568 = local read "Buffer-C2 PickUp \nFlow Rate (ul/min)"() -> (w3946:dbl)
                            n3569 = local read "Buffer-C2 Pumping\nResolution"() -> (w3945:T2)
                            n3570 = local read "VISA Refnum in\nfor Pump"() -> (w3948:refnum<visa-resource-name>)
                            n3571 = local read "Buffer-C2 Volume \nto be Pumped"() -> (w3944:dbl)
                            n3572 = local read "Volume of Syringe"() -> (w3947:dbl)
                            n3573 = call "RPickUp(SubVI).vi"("Volume to be picked up"=w3944, "Volume of Syringe"=w3947, "Resolution of PickUP"=w3945, "PickUp Flow Rate (ul/min)"=w3946, "VISA Refnum in"=w3948) -> ()  [unwired: 6 in, 1 out]
                            n3574 = local write "SEC On"(TRUE ("SEC On")) -> ()
                          }
                          frame #22 {
                            n3575 = local read "Stopper that ends \nthe main loops"() -> (w3949:bool)
                            n3576 = local read "VISA Refnum in\nfor Pump"() -> (w3950:refnum<visa-resource-name>)
                            n3577 = case shown="True" w3949 {
                              frame False {
                              }
                              frame True {
                                n3578 = local read "VISA Refnum in\nfor Pump"() -> (w3951:refnum<visa-resource-name>)
                                n3579 = call "HardStopCurrentProcess (SubVI).vi"("VISA Refnum in"=w3951) -> ()  [unwired: 11 in]
                              }
                            }
                            n3580 = call "ProcessCompletionWaiter (SubVI).vi"("VISA Refnum in"=w3950) -> ()  [unwired: 11 in]
                          }
                          frame #23 {
                            # "Reads the initial Plunger Position for computing the volume dispensed"
                            n3581 = local read "VISA Refnum in\nfor Pump"() -> (w3953:refnum<visa-resource-name>)
                            n3582 = call "AbsolutePlungerPosition (SubVI).vi"("VISA Refnum in"=w3953) -> ("Plunger Position"=w3952:i32)  [unwired: 10 in]
                            n3583 = local write "Initial Plunger Position"(w3952) -> ()
                          }
                          frame #24 {
                            # "Switch to Port-10"
                            # "Port-10 of the pump is conncted to column-2 of chip"
                            n3584 = local read "VISA Refnum in\nfor Pump"() -> (w3955:refnum<visa-resource-name>)
                            n3585 = call "PortChanger (SubVI).vi"("Port Number"="10", "VISA Refnum in"=w3955) -> ()  [unwired: 10 in]
                          }
                          frame #25 {
                            n3586 = local read "Stopper that ends \nthe main loops"() -> (w3956:bool)
                            n3587 = local read "VISA Refnum in\nfor Pump"() -> (w3957:refnum<visa-resource-name>)
                            n3588 = case shown="True" w3956 {
                              frame False {
                              }
                              frame True {
                                n3589 = local read "VISA Refnum in\nfor Pump"() -> (w3958:refnum<visa-resource-name>)
                                n3590 = call "HardStopCurrentProcess (SubVI).vi"("VISA Refnum in"=w3958) -> ()  [unwired: 11 in]
                              }
                            }
                            n3591 = call "ProcessCompletionWaiter (SubVI).vi"("VISA Refnum in"=w3957) -> ()  [unwired: 11 in]
                          }
                          frame #26 {
                            # "Keeps the AMF valve after column-1 open and valve after column-2 closed"
                            n3592 = local read "Buffer-C2 Dispense\nFlow Rate (ul/min)"() -> (w3971:dbl)
                            n3593 = local read "Buffer-C2 Pumping\nResolution"() -> (w3970:T2)
                            n3594 = local read "VISA Refnum in\nfor Pump"() -> (w3973:refnum<visa-resource-name>)
                            n3595 = local write "Pause Data Collection"(FALSE ("Pause Data Collection")) -> ()
                            n3596 = local read "Volume of Syringe"() -> (w3972:dbl)
                            n3597 = call "GoToAbsolutePosition(SubVI).vi"("Absolute Volume Position in Syringe (in ul)"=0.0 ("Volume to be Dispensed"), "Volume of Syringe"=w3972, "Resolution of Pumping"=w3970, "Flow Rate (ul/min)"=w3971, "VISA Refnum in"=w3973) -> ()  [unwired: 6 in, 1 out]
                            n3598 = local read "VISA Refnum in\nfor Valve"() -> (w3967:refnum<visa-resource-name>)
                            n3599 = local read "External Valve \nOPEN"() -> (w3966:string)
                            n3600 = local write "Valve V1 Open"(FALSE ("Valve V1 Open")) -> ()
                            n3601 = local write "Valve V2 Open"(TRUE ("Valve V2 Open")) -> ()
                            n3602 = local write "Valve V3 Open"(TRUE ("Valve V3 Open")) -> ()
                            n3603 = local write "Valve V4 Open"(FALSE ("Valve V4 Open")) -> ()
                            n3604 = call "PortChanger_Valve (SubVI).vi"("Port Number"=w3966, "VISA Refnum in"=w3967) -> ()  [unwired: 10 in]
                            n3605 = local write "Valve V5 Open"(FALSE ("Valve V5 Open")) -> ()
                            n3606 = local write "Valve V6 Open"(FALSE ("Valve V6 Open")) -> ()
                            n3607 = local write "Valve V7 Open"(FALSE ("Valve V7 Open")) -> ()
                          }
                          frame #27 {
                            n3608 = local read "Initial Plunger Position"() -> (w3977:dbl)
                            n3609 = local read "Buffer-C2 Pumping\nResolution"() -> (w3976:T2)
                            n3610 = local read "VISA Refnum in\nfor Pump"() -> (w3978:refnum<visa-resource-name>)
                            n3611 = local read "Volume of Syringe"() -> (w3975:dbl)
                            n3612 = while {
                              tunnel: w3977 -> [w3984]
                              tunnel: w3978 -> [w3983]
                              tunnel: w3976 -> [w3982]
                              tunnel: w3975 -> [w3981]
                              stop <- w3979 stop-if-true
                              n3613 = Wait (ms)(milliseconds to wait=u32 100) -> ()  [unwired: 1 out]
                              n3614 = stacked-sequence {
                                tunnel: w3984 -> [w3990 _]
                                tunnel: w3983 -> [w3989 w4016]
                                tunnel: w3982 -> [w3988 _]
                                tunnel: w3981 -> [w3987 _]
                                tunnel: [_ w4012] -> w3979
                                frame #0 {
                                n3615 = call "AbsolutePlungerPosition (SubVI).vi"("VISA Refnum in"=w3989) -> ("Plunger Position"=w3986:i32)  [unwired: 10 in]
                                n3616 = case shown="\"Standard Pumping\", Default" w3988 {
                                tunnel: w3990 -> [w3995 w4004]
                                tunnel: w3986 -> [w3996 w4003]
                                tunnel: [w3994 w4001] -> w3985
                                tunnel: w3987 -> [w3993 w4002]
                                frame "Standard Pumping", Default {
                                n3617 = Subtract(x=w3995, y=w3996) -> (x-y=w3992:dbl)
                                n3618 = Absolute Value(x=w3992) -> (abs(x)=w3991:dbl)
                                n3619 = Multiply(x=w3991, y=w3993) -> (x*y=w3998:dbl)
                                n3620 = Divide(x=w3998, y=3000.0) -> (x/y=w3994:dbl)
                                }
                                frame "High Resolution Pumping" {
                                n3621 = Subtract(x=w4004, y=w4003) -> (x-y=w4000:dbl)
                                n3622 = Absolute Value(x=w4000) -> (abs(x)=w3999:dbl)
                                n3623 = Multiply(x=w3999, y=w4002) -> (x*y=w4006:dbl)
                                n3624 = Divide(x=w4006, y=24000.0) -> (x/y=w4001:dbl)
                                }
                                }
                                n3625 = local write "Volume being Injected \nin this process"(w3985) -> ()
                                }
                                frame #1 {
                                n3626 = local read "Stopper that ends \nthe main loops"() -> (w4013:bool)
                                n3627 = local read "Divert Buffer-C \ninto Column-2"() -> (w4014:bool)
                                n3628 = local read "Volume being Injected \nin this process"() -> (w4011:dbl)
                                n3629 = call "LSPOneStatus (SubVI).vi"("VISA Refnum in"=w4016) -> ("read buffer"=w4018:string)  [unwired: 10 in]
                                n3630 = call <vilib>:"Trim Whitespace.vi"("string"=w4018) -> ("trimmed string"=w4017:string)  [unwired: 1 in]
                                n3631 = Equal?(x=w4017, y="/0`\u0003") -> (x = y?=w4015:bool)
                                n3632 = Or(x=w4014, y=w4013) -> (x .or. y?=w4009:bool)
                                n3633 = Greater Or Equal?(x=w4011, y=2.0) -> (x >= y?=w4008:bool)
                                n3634 = Or(x=w4009, y=w4008) -> (x .or. y?=w4007:bool)
                                n3635 = Or(x=w4015, y=w4007) -> (x .or. y?=w4012:bool)
                                }
                              }
                            }
                            n3636 = local read "Stopper that ends \nthe main loops"() -> (w3974:bool)
                            n3637 = case shown="True" w3974 {
                              frame False {
                              }
                              frame True {
                                n3638 = local read "VISA Refnum in\nfor Pump"() -> (w4020:refnum<visa-resource-name>)
                                n3639 = call "HardStopCurrentProcess (SubVI).vi"("VISA Refnum in"=w4020) -> ()  [unwired: 11 in]
                              }
                            }
                          }
                          frame #28 {
                            # "Keeps the on-chip valves V4, V5 and V7 open"
                            # "Keeps the AMF valve after column-1 closed and valve after column-2 open"
                            n3640 = local write "Divert Buffer-C \ninto Column-2"(FALSE ("Divert Buffer-C \ninto Column-2")) -> ()
                            n3641 = local read "VISA Refnum in\nfor Pump"() -> (w4025:refnum<visa-resource-name>)
                            n3642 = local read "External Valve \nCLOSED"() -> (w4024:string)
                            n3643 = local write "Valve V3 Open"(FALSE ("Valve V3 Open")) -> ()
                            n3644 = local write "Valve V2 Open"(FALSE ("Valve V2 Open")) -> ()
                            n3645 = local write "Valve V1 Open"(FALSE ("Valve V1 Open")) -> ()
                            n3646 = local write "Valve V4 Open"(TRUE ("Valve V4 Open")) -> ()
                            n3647 = call "PortChanger_Valve (SubVI).vi"("Port Number"=w4024, "VISA Refnum in"=w4025) -> ()  [unwired: 10 in]
                            n3648 = local write "Valve V5 Open"(TRUE ("Valve V5 Open")) -> ()
                            n3649 = local write "Valve V6 Open"(FALSE ("Valve V6 Open")) -> ()
                            n3650 = local write "Valve V7 Open"(TRUE ("Valve V7 Open")) -> ()
                          }
                          frame #29 {
                            n3651 = local read "Initial Plunger Position"() -> (w4034:dbl)
                            n3652 = local read "Buffer-C2 Pumping\nResolution"() -> (w4033:T2)
                            n3653 = local read "VISA Refnum in\nfor Pump"() -> (w4035:refnum<visa-resource-name>)
                            n3654 = local read "Volume of Syringe"() -> (w4032:dbl)
                            n3655 = while {
                              tunnel: w4034 -> [w4041]
                              tunnel: w4035 -> [w4040]
